vi "Keithley DMM6500 DAQ6500 Series Measuring DCV With High Accuracy DCV.vi"() -> ()   [LabVIEW 2023]
doc: "This example shows how to get high accuracy DC voltage measurement."
uses:
  <instrlib>/Keithley DMM6500 DAQ6500 Series/Public/Data/Read (Single Point).vi
  <instrlib>/Keithley DMM6500 DAQ6500 Series/Keithley DMM6500 DAQ6500 Series.lvlib
panel:
  in  "Enable Average Filter (F: Disable)":bool
  in  "Input Impedance (0: 10Mohm)":i32(ring) items=["10Mohm", "Auto"]
  in  "Auto Zero (0: Enable)":u32(ring) items=["Enable", "Disable", "Once"]
  in  "Auto Range (T: Enable)":bool=TRUE
  in  "Average Filter Type (0: Repeat)":i32(ring) items=["Repeat", "Moving"]
  in  "Power Line Cycle (1)":dbl=10.0
  out "Measurement":dbl
  in  "Average Count (10)":u32=10
  in  "Manual Range (0)":dbl=10.0
  in  "Channel List (\"101\")":string="101"
  in  "VISA resource name":refnum<visa-resource-name>
  # "(c) 2018-2022 National Instruments.  ALL RIGHTS RESERVED."
  # "This example application demonstrates how to use a DMM6500 or DAQ6500 Series to make a high-accuracy DC voltage measurement from the front or rear terminals. \nIf it's for DMM the Channel List control will take no effect."
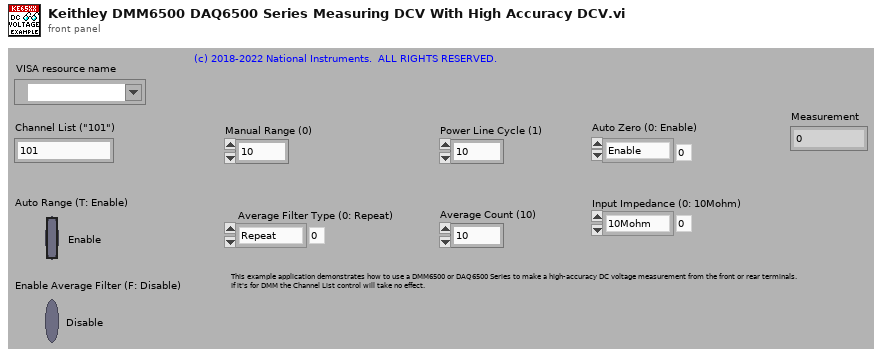
[diagram p1: front panel]
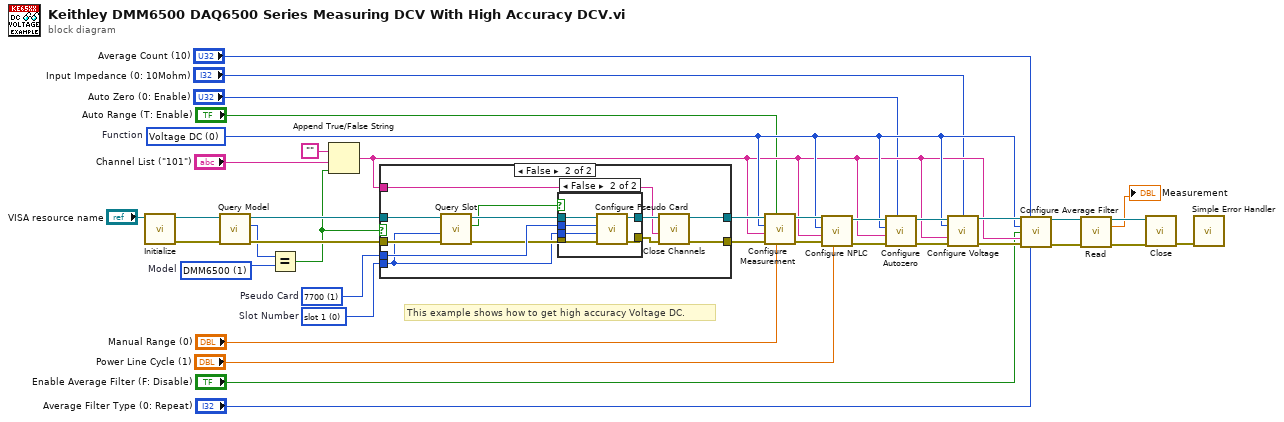
[diagram p0: block diagram]
diagram:
  w36 = 0 items=["slot 1", "slot 2"]  # Slot Number
  w37 = 1 items=["0", "7700", "7701", "7702", "7703", "7705", "7706", "7707", "7708", "7709", "7710", "7711", "7712"]  # Pseudo Card
  w10 = 0 items=[" Voltage DC", "Voltage AC", "Current DC", "Current AC", "Resistance", "4-wire Resistance", "Diode", "Capacitance", "Temperature", "Continuity", "Frequency", "Period", "Voltage Ratio", "Digitize Voltage", "Digitize Current"]  # Function
  w11 = 1 items=["", "DMM6500", "DAQ6510"]  # Model
  # "This example shows how to get high accuracy Voltage DC."
  n1 = call <instrlib>:"Initialize.vi"("VISA resource name"="VISA resource name") -> ("error out"=w14:errorcluster, "VISA resource name out"=w16:refnum<visa-resource-name>)  [unwired: 9 in]
  n2 = call <instrlib>:"Query Model.vi"("error in (no error)"=w14, "VISA resource name"=w16) -> ("error out"=w13:errorcluster, "Model"=w12:i32, "VISA resource name out"=w15:refnum<visa-resource-name>)  [unwired: 7 in]
  n3 = Equal?(x=w12, y=w11) -> (x = y?=w6:bool)
  n4 = Append True/False String(1:w6, 2:"Channel List (\"101\")", 3:"") -> (0:w9:string)  [unwired: 1 in]
  n5 = case shown="False" w6 {
    tunnel: w37 -> [_ w52]
    tunnel: w36 -> [_ w42]
    tunnel: w15 -> [w40 w51]
    tunnel: w13 -> [w39 w44]
    tunnel: [w40 w49] -> w20
    tunnel: [w39 w47] -> w18
    tunnel: w9 -> [_ w46]
    frame True {
    }
    frame False {
      n6 = call <instrlib>:"Query Slot.vi"("error in (no error)"=w44, "Slot Number(0: slot 1)"=w42, "VISA resource name"=w51) -> ("error out"=w43:errorcluster, "Real Card In Slot"=w41:bool, "VISA resource name out"=w45:refnum<visa-resource-name>)  [unwired: 6 in]
      n7 = case shown="False" w41 {
        tunnel: w52 -> [_ w60]
        tunnel: [w54 w59] -> w50
        tunnel: [w53 w58] -> w48
        tunnel: w45 -> [w54 w57]
        tunnel: w43 -> [w53 w56]
        tunnel: w42 -> [_ w55]
        frame True {
        }
        frame False {
          n8 = call <instrlib>:"Configure Pseudo Card.vi"("error in (no error)"=w56, "Slot Number (0: slot1)"=w55, "Pseudo Card (0:No pseudocard)"=w60, "VISA resource name"=w57) -> ("error out"=w58:errorcluster, "VISA resource name out"=w59:refnum<visa-resource-name>)  [unwired: 6 in]
        }
      }
      n9 = call <instrlib>:"Close Channels.vi"("error in (no error)"=w48, "Channel List(\"\")"=w46, "VISA resource name"=w50) -> ("error out"=w47:errorcluster, "VISA resource name out"=w49:refnum<visa-resource-name>)  [unwired: 7 in]
    }
  }
  n10 = call <instrlib>:"Configure Measurement.vi"("Manual Range (1)"="Manual Range (0)", "Auto Range (T: Enable)"="Auto Range (T: Enable)", "error in (no error)"=w18, "Channel List(\"\")"=w9, "Function (0: Voltage DC)"=w10, "VISA resource name"=w20) -> ("error out"=w17:errorcluster, "VISA resource name out"=w19:refnum<visa-resource-name>)  [unwired: 4 in]
  n11 = call <instrlib>:"Configure NPLC.vi"("Power Line Cycle (1)"="Power Line Cycle (1)", "error in (no error)"=w17, "Channel List(\"\")"=w9, "Function (0: Voltage DC)"=w10, "VISA resource name"=w19) -> ("error out"=w32:errorcluster, "VISA resource name out"=w33:refnum<visa-resource-name>)  [unwired: 5 in]
  n12 = call <instrlib>:"Configure Autozero.vi"("Auto Zero (0: Enable)"="Auto Zero (0: Enable)", "error in (no error)"=w32, "Channel List(\"\")"=w9, "Function (0: Voltage DC)"=w10, "VISA resource name"=w33) -> ("error out"=w30:errorcluster, "VISA resource name out"=w31:refnum<visa-resource-name>)  [unwired: 5 in]
  n13 = call <instrlib>:"Configure Voltage.vi"("VISA resource name"=w31, "Input Impedance (0: 10Mohm)"="Input Impedance (0: 10Mohm)", "Function (0: Voltage DC)"=w10, "Channel List(\"\")"=w9, "error in (no error)"=w30) -> ("VISA resource name out"=w29:refnum<visa-resource-name>, "error out"=w28:errorcluster)  [unwired: 9 in]
  n14 = call <instrlib>:"Configure Average Filter.vi"("VISA resource name"=w29, "Count (10)"="Average Count (10)", "Function (0: Voltage DC)"=w10, "Enable Average Filter (F: Disable)"="Enable Average Filter (F: Disable)", "Channel List (\"\")"=w9, "error in (no error)"=w28, "Average Filter Type (0: Repeat)"="Average Filter Type (0: Repeat)") -> ("VISA resource name out"=w26:refnum<visa-resource-name>, "error out"=w25:errorcluster)  [unwired: 7 in]
  n15 = call-poly <instrlib>:"Read.vi"("VISA resource name"=w26, "error in (no error)"=w25) -> ("VISA resource name out"=w23:refnum<visa-resource-name>, "Measurement"=→"Measurement":dbl, "error out"=w24:errorcluster)  [unwired: 11 in]
  n16 = call <instrlib>:"Close.vi"("error in (no error)"=w24, "VISA resource name"=w23) -> ("error out"=w38:errorcluster)  [unwired: 9 in]
  n17 = call <vilib>:"Simple Error Handler.vi"("error in (no error)"=w38) -> ()  [unwired: 4 in, 5 out]
